vi "fact using reg.vi"() -> ()   [LabVIEW 2022 SP3]
panel:
  out "Numeric":dbl
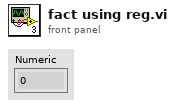
[diagram p1: front panel]
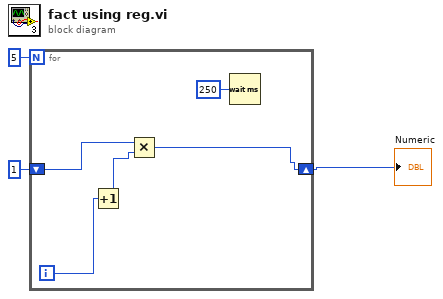
[diagram p0: block diagram]
diagram:
  n1 = for {
    N: 5 -> [_]
    shift-right: [w6] -> w2
    shift-left: 1 -> [w5]
    i -> [w8]
    n2 = Increment(x=w8) -> (x+1=w7:i32)
    n3 = Multiply(x=w5, y=w7) -> (x*y=w6:i32)
    n4 = Wait (ms)(milliseconds to wait=u32 250) -> ()  [unwired: 1 out]
  }
  "Numeric" <- w2
